vi "TW Convert Top Level.vi"() -> ()   [LabVIEW 2021, in "Plugin Generator.lvlib"]
uses:
  Plugin Generator.lvlib
  <vilib>/CIF Foundation/CIF LabVIEW Scripting/LV Scripting/Typedef/Icon Overlay.ctl
  <vilib>/CIF Foundation/CIF Core/Channels/ChannelRegistrar/typedef/Channel Definition for Scripting.ctl
  <vilib>/CIF Foundation/CIF Channels Core/CIFChannels/Typedef/Direction.ctl
  <vilib>/CIF Foundation/CIF Core/Channels/ChannelRegistrar/typedef/Registered Channel Types.ctl
  <vilib>/CIF Foundation/CIF LabVIEW Scripting/LV Scripting/LV Scripting Utilities.lvlib
  <vilib>/CIF Foundation/CIF Channels Core/CIFChannels/CIFChannels.lvclass
  <vilib>/CIF Foundation/CIF Core/Channels/ChannelRegistrar/ChannelRegistrar.lvlib
panel:
  in  "Channels to Create":T1[](array[typedef])
  in  "Icon Overlay":T4={"Text"="", "Background color"=7208704, "Text color"=0}
  out "error out":errorcluster
  in  "New Name":string="CIFRocks"
  in  "Template Project Path":path=path "D:/dev/Plugins/ROCK - Copy/Tests/Template Interactive Test.lvproj"
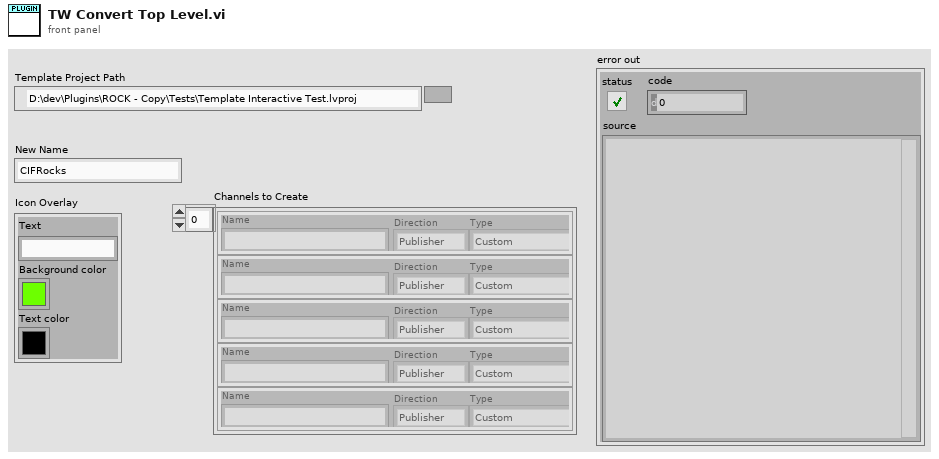
[diagram p1: front panel]
types:
  T1 = typedef "ChannelRegistrar.lvlib/Channel Definition for Scripting.ctl" = cluster{"Name":string, "Direction":T2, "Type":T3}
  T2 = typedef "CIFChannels.lvclass/Direction.ctl" = enum16{"Publisher", "Subscriber"}
  T3 = typedef "ChannelRegistrar.lvlib/Registered Channel Types.ctl" = enum16{"Custom", "Double_Tag", "I64_Tag", "U64_Tag", "U8_FIFO", "CAN_FIFO", "L2Enet_FIFO", "DAQ_FIFO", "Universal_FIFO", "String_Tag"}
  T4 = typedef "LV Scripting Utilities.lvlib/Icon Overlay.ctl" = cluster{"Text":string, "Background color":u32, "Text color":u32}
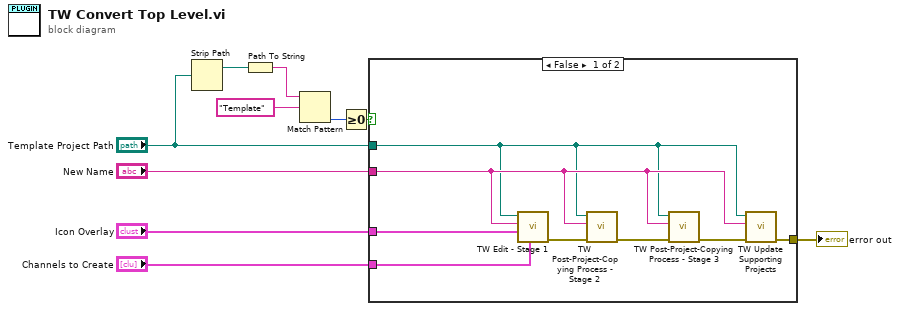
[diagram p0: block diagram]
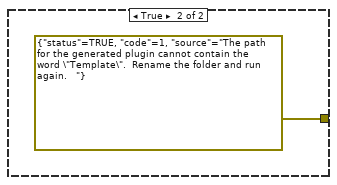
[diagram p2: hidden frame]
diagram:
  n1 = Strip Path(path="Template Project Path") -> (stripped path=w7:path)  [unwired: 1 out]
  n2 = Path To String(path=w7) -> (string=w6:string)
  n3 = Match Pattern(string=w6, regular expression="Template") -> (offset past match=w4:i32)  [unwired: 1 in, 3 out]
  n4 = Greater Or Equal To 0?(x=w4) -> (x >= 0?=w3:bool)
  n5 = case shown="False" w3 {
    tunnel: [w15 errorcluster {"status"=TRUE, "code"=1, "source"="The path for the generated plugin cannot contain the word \"Template\".  Rename the folder and run again.   "} ("error out")] -> w10
    tunnel: "New Name" -> [w14 _]
    tunnel: "Template Project Path" -> [w13 _]
    tunnel: "Icon Overlay" -> [w12 _]
    tunnel: "Channels to Create" -> [w11 _]
    frame False {
      n6 = call "TW Edit - Stage 1.vi"("Channels to Create"=w11, "Icon Overlay"=w12, "New Subname"=w14, "Template Project Path"=w13) -> ("error out"=w18:errorcluster)  [unwired: 7 in]
      n7 = call "TW Post-Project-Copying Process - Stage 2.vi"("error in"=w18, "New Subname"=w14, "Template Project Path"=w13) -> ("error out"=w17:errorcluster)  [unwired: 8 in]
      n8 = call "TW Post-Project-Copying Process - Stage 3.vi"("error in"=w17, "New Subname"=w14, "Template Project Path"=w13) -> ("error out"=w16:errorcluster)  [unwired: 8 in]
      n9 = call "TW Update Supporting Projects.vi"("error in (no error)"=w16, "New Name"=w14, "Template Project Path"=w13) -> ("error out"=w15:errorcluster)  [unwired: 8 in]
    }
    frame True {
    }
  }
  "error out" <- w10
